vi "Sign Changes.vi"(8 "x1":dbl, 9 "x0":dbl, 11 "f":dbl[](array[numeric])) -> (3 "number of roots":i32)   [LabVIEW 2018, in "NI_AALPro.lvlib"]
doc: "From ../labview/vi.lib/gmath/zeros.llb."
uses:
  NI_AALPro.lvlib
  1D Polynomial Evaluation (DBL).vi
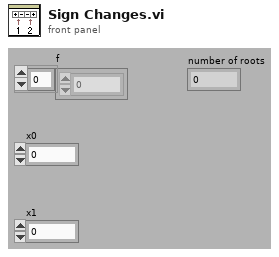
[diagram p1: front panel]
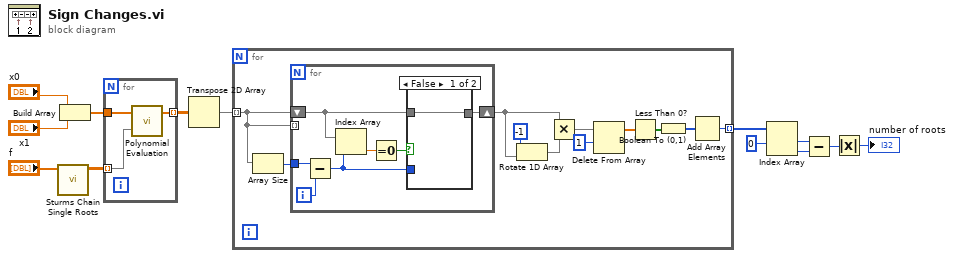
[diagram p0: block diagram]
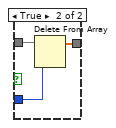
[diagram p2: hidden frame]
diagram:
  n1 = call "Sturms Chain Single Roots.vi"("f"="f") -> ("sequence of polynomials"=w13:dbl[][])  [unwired: 10 in]
  n2 = Build Array("x0", "x1") -> (w6:dbl[])
  n3 = for {
    tunnel: w13 -> [w15] mode=indexing
    tunnel: [w14] -> w12 mode=indexing
    tunnel: w6 -> [w16]
    n4 = call-poly "Polynomial Evaluation.vi"("P(x)"=w15, "A"=w16) -> ("P(A)"=w14:dbl[])  [unwired: 1 out]
  }
  n5 = Transpose 2D Array(2D array=w12) -> (transposed array=w11:dbl[][])
  n6 = for {
    tunnel: w11 -> [w18] mode=indexing
    tunnel: [w19] -> w10 mode=indexing
    n7 = Array Size(array=w18) -> (size(s)=w17:i32)
    n8 = for {
      shift-right: [w31] -> w26
      shift-left: w18 -> [w32]
      tunnel: w18 -> [_] mode=indexing
      tunnel: w17 -> [w29]
      i -> [w30]
      n9 = Subtract(x=w29, y=w30) -> (x-y=w28:i32)
      n10 = Index Array(array=w32, index=w28) -> (element=w34:dbl)
      n11 = Equal To 0?(x=w34) -> (x = 0?=w33:bool)
      n12 = case shown="False" w33 {
        tunnel: w32 -> [w35 w38]
        tunnel: [w35 w37] -> w31
        tunnel: w28 -> [_ w36]
        frame False {
        }
        frame True {
          n13 = Delete From Array(array=w38, index=w36) -> (array with subset deleted=w37:dbl[])  [unwired: 1 in, 1 out]
        }
      }
    }
    n14 = Rotate 1D Array(1:w26, 2:-1) -> (0:w25:dbl[])
    n15 = Multiply(x=w26, y=w25) -> (x*y=w24:dbl[])
    n16 = Delete From Array(array=w24, length=1) -> (array with subset deleted=w22:dbl[])  [unwired: 1 in, 1 out]
    n17 = Less Than 0?(x=w22) -> (x < 0?=w21:bool[])
    n18 = Boolean To (0,1)(Boolean=w21) -> (0, 1=w20:i16[])
    n19 = Add Array Elements(numeric array=w20) -> (sum=w19:i16)
  }
  n20 = Index Array(array=w10, index #1=0) -> (element #1=w8:i16, element #2=w5:i16)  [unwired: 1 in]
  n21 = Subtract(x=w8, y=w5) -> (x-y=w7:i16)
  n22 = Absolute Value(x=w7) -> (abs(x)=→"number of roots":i16)
